vi "Color_movement.vi"(2 "Color Number":u8=4, 3 "moveLog(Row, Col.)":i32[][](array[numeric]), 4 "bitmap":i32[][](array[numeric])) -> (1 "Colored bitmap":i32[][](array[numeric]))   [LabVIEW 2016]
panel:
  # "4 : red\n7:green"
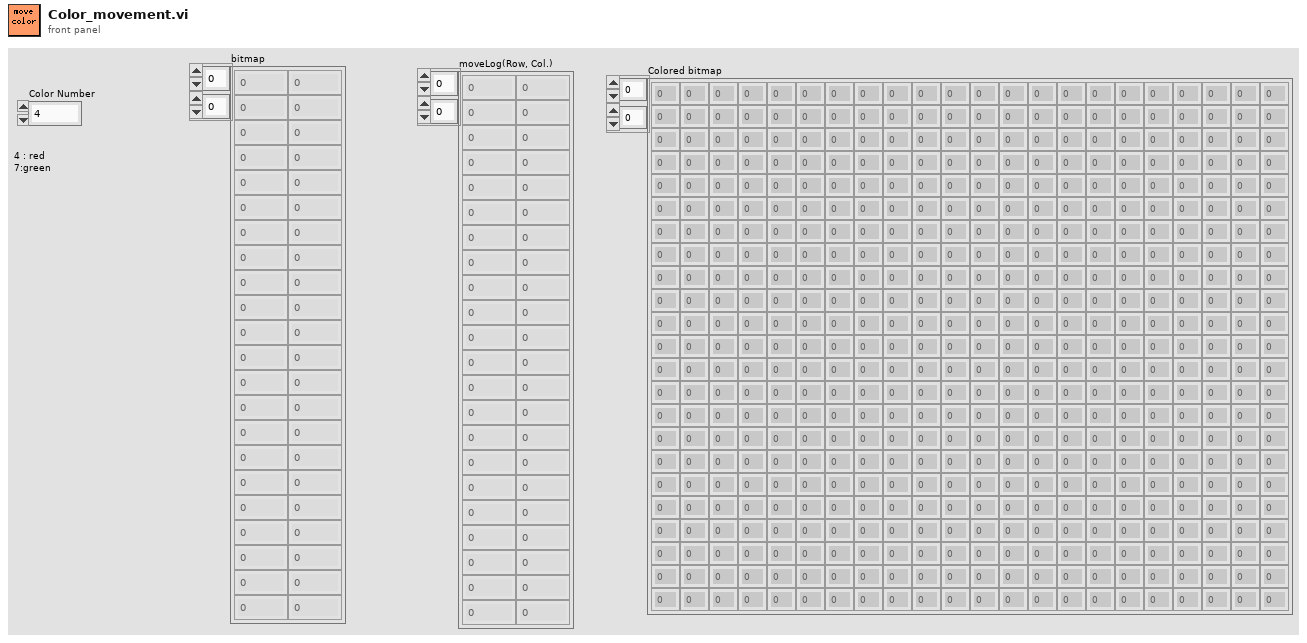
[diagram p1: front panel]
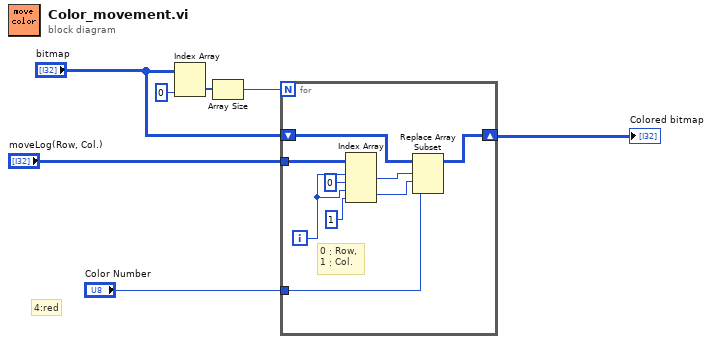
[diagram p0: block diagram]
diagram:
  # "4:red"
  n1 = Index Array(array="bitmap", index (col)=0 ("無効な指標 （列）")) -> (element=w4:i32[])  [unwired: 1 in]
  n2 = Array Size(array=w4) -> (size(s)=w2:i32)
  n3 = for {
    N: w2 -> [_]
    tunnel: "moveLog(Row, Col.)" -> [w16]
    shift-right: [w10] -> w5
    shift-left: "bitmap" -> [w9]
    tunnel: "Color Number" -> [w8]
    i -> [w14]
    # "0：Row,\n1：Col."
    n4 = Index Array(array=w16, index (row) #1=w14, index (col) #1=0 ("無効な指標 （列）"), index (row) #2=w14, index (col) #2=1 ("無効な指標 （列）")) -> (element #1=w12:i32, element #2=w11:i32)
    n5 = Replace Array Subset(array=w9, new element=w8, index (row)=w12, index (col)=w11) -> (w10:i32[][])
  }
  "Colored bitmap" <- w5
